vi "AlazarRead.vi"(0 "DeviceIn":i32, 1 "Digitizer Settings":T1={"Digitizer delay (us) "=18.666667, "rf points per line"=4000, "lines per plane"=139, "Samp Rate (Hz)"=100000000.0, "Additional dig delay (us)"=0.0, "Voltage Scale"=0.4, "Pre-Looks"=0, "Offset delay (us)"=2.0, "bits A/D"=0, "Avg Num"=1, "DigTimeOut"=5.0, "Rel Dig Delay"=0.0, "Dig Ch"=0, "LeCroyCluster"={"LeCroy Channels"=[TRUE, FALSE, FALSE, FALSE], "LC read pt offset"=0.0, "Sweep Avg"=FALSE}, "Main Digitizer"=enum."NI Digitizer", "Dig Config"=enum."Single channel", "Digitizer ID Cluster"={"Acqiris/Alazar/SP ID"=[], "NI Instr Handles"=[], "LeCroy VISA"="", "GaGe Handle"={"Handle"=0, "Sample size"=0, "Resolution"=0, "Offset"=0, "Channels"=0, "Boards"=0}, "ATS Ref"="ATS9350", "Acqiris Address"=["PCI::INSTR0"], "ADQRef"=refnum, "adq_cu_ptr"=refnum}, "Trigger Settings"={"Trig Source"=1, "Trig Coupling"=0, "Trig Slope"=0, "Level (mV)"=1500.0}, "Bulk Acq"=FALSE, "Bulk Start Indexes"=[], "Data Ref RF"=refnum, "NI ID/Channel"=[], "Total Dig CH"=1, "Xtra Ann Trig delay (us)"=10.0, "Fix Z Delay?"=FALSE, "One Way Transmission?"=FALSE, "Data Ref Log"=refnum} {"Trigger Settings"."Trig Slope" items=["Positive", "Negative"]; "Trigger Settings"."Level (mV)" format="%.2f"; "Trigger Settings"."Trig Coupling" items=["DC 1 MOhm", "AC 1 MOhm", "DC 50 Ohm", "AC 50 Ohm"]; "Trigger Settings"."Trig Source" items=["Chan 1", "External"]; "Rel Dig Delay" format="%.2f"; "DigTimeOut" format="%.2f"; "Avg Num" min=1; "Offset delay (us)" format="%.2f"; "Additional dig delay (us)" format="%.2f"; "Digitizer delay (us)" format="%.2f"}, 5 "Channel":T5, 9 "RecordIn":u32=1, 11 "ReadSamples":T6) -> (3 "Clock (s)":dbl format="%.2p", 4 "DeviceOut":i32, 6 "TimeStamp (s)":dbl format="%.2p", 8 "Voltage Scaling":dbl, 10 "Presize (s)":dbl format="%.2p", 14 "Binary Data":i16[](array[numeric]), 15 "Return Code":u32)   [LabVIEW 2022 SP3]
doc: "_____AlazarTech, Scope_____\n\nConfigure the capture clock circuitry."
uses:
  C:/AlazarTech/ATS-VI/6.2.0/ATS_ctl/Device_Ctrl.ctl
  ATS_ReadSamples.ctl
  C:/AlazarTech/ATS-VI/6.2.0/ATS_ctl/ATS_Channel.ctl
  -DigitizerRoutines/DigitizerSettings.ctl
  -DigitizerRoutines/DigitizerID.ctl
  -DigitizerRoutines/Digitizer.ctl
  -DigitizerRoutines/DigConfig.ctl
  C:/Windows/System32/ADQAPI_dotNet_helper.dll
panel:
  out "Waveform Graph":i16[](graph)
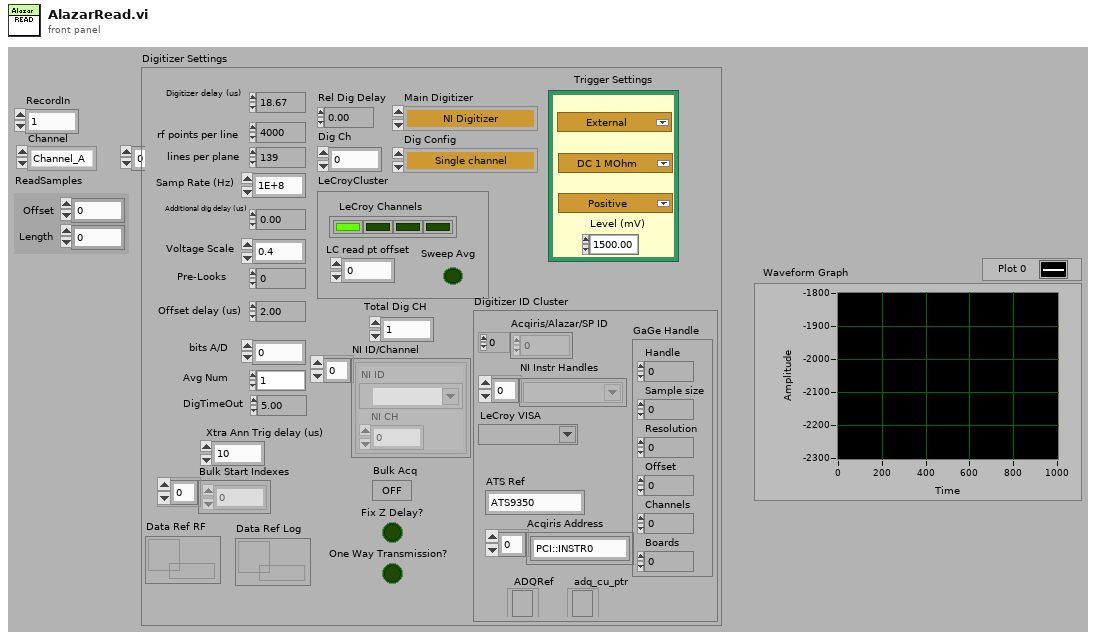
[diagram p1: front panel]
types:
  T1 = typedef "DigitizerSettings.ctl" = cluster{"Digitizer delay (us) ":dbl, "rf points per line":i32, "lines per plane":i32, "Samp Rate (Hz)":dbl, "Additional dig delay (us)":dbl, "Voltage Scale":dbl, "Pre-Looks":i32, "Offset delay (us)":dbl, "bits A/D":i8, "Avg Num":i32, "DigTimeOut":sgl, "Rel Dig Delay":sgl, "Dig Ch":i32, "LeCroyCluster":cluster{"LeCroy Channels":bool[], "LC read pt offset":dbl, "Sweep Avg":bool}, "Main Digitizer":T2, "Dig Config":T3, "Digitizer ID Cluster":T4, "Trigger Settings":cluster{"Trig Source":u16, "Trig Coupling":u16, "Trig Slope":u16, "Level (mV)":dbl}, "Bulk Acq":bool, "Bulk Start Indexes":i32[], "Data Ref RF":refnum<data-value>, "NI ID/Channel":cluster{"NI ID":refnum<k15>, "NI CH":i32}[], "Total Dig CH":i32, "Xtra Ann Trig delay (us)":dbl, "Fix Z Delay?":bool, "One Way Transmission?":bool, "Data Ref Log":refnum<data-value>}
  T2 = typedef "Digitizer.ctl" = enum16{"Acqiris Digitizer", "NI Digitizer", "LeCroy", "GaGe", "AlazarTech", "No Digitizer", "Teledyne"}
  T3 = typedef "DigConfig.ctl" = enum16{"Single channel", "2 Chans w/ 2 Acqiris", "2 Chans w/ 1 Acqiris", "5-CH Pulser New", "5-CH pulser w/ ann array", "5-pass style ann array", "Empty"}
  T4 = typedef "DigitizerID.ctl" = cluster{"Acqiris/Alazar/SP ID":u32[], "NI Instr Handles":refnum<k15>[], "LeCroy VISA":refnum<visa-resource-name>, "GaGe Handle":cluster{"Handle":u32, "Sample size":u32, "Resolution":i32, "Offset":i32, "Channels":u32, "Boards":u32}, "ATS Ref":string, "Acqiris Address":string[], "ADQRef":refnum<k24>, "adq_cu_ptr":refnum<k24>}
  T5 = typedef "ATS_Channel.ctl" = enum16{"Channel_A", "Channel_B", "Channel_C", "Channel_D"}
  T6 = typedef "ATS_ReadSamples.ctl" = cluster{"Offset":i32, "Length":u32}
  T7 = typedef "Device_Ctrl.ctl" = enum16{"Status", "About", "Arm", "ForceTrig", "Abort", "Initialize", "Init (NoPreset)", "Info", "Close", "Calibrate", "SetManually", "LED_ON", "LED_OFF"}
  T8 = typedef "Device_Info.ctl" = cluster{"Handle":u32, "Board":string, "CPLD":string, "MemorySize":u32, "SampleSize":u8, "ID":i32, "High_Memory":bool, "Chan/Board":u8}
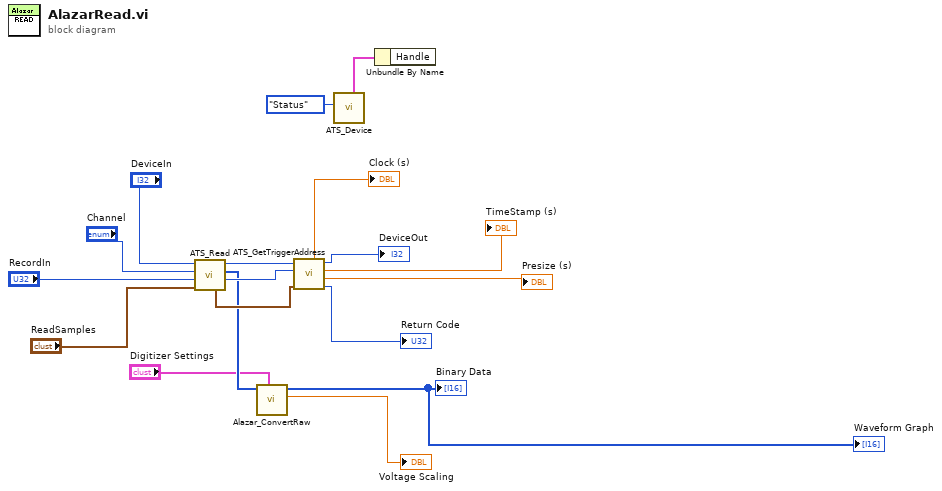
[diagram p0: block diagram]
diagram:
  n1 = call "ATS_Read.vi"("ReadSamples"="ReadSamples", "RecordIn"="RecordIn", "Channel"="Channel", "DeviceIn"="DeviceIn") -> ("RecordOut"=w11:u32, "Buffer"=w4:u16[], "DeviceOut"=w15:i32, "ReadSamples_Out"=w12:T6)  [unwired: 3 in, 1 out]
  n2 = call "Alazar_ConvertRaw.vi"("Digitizer Settings"="Digitizer Settings", "Buffer"=w4) -> ("Voltage multiplier"=→"Voltage Scaling":dbl, "Array"=→"Binary Data" →"Waveform Graph":i16[])  [unwired: 8 in]
  n3 = call "ATS_GetTriggerAddress.vi"("ReadSamples"=w12, "Record"=w11, "DeviceIn"=w15) -> ("Return Code"=→"Return Code":u32, "Presize (s / clk)"=→"Presize (s)":dbl, "TimeStamp (s / clk)"=→"TimeStamp (s)":dbl, "DeviceOut"=→"DeviceOut":i32, "Clock (s / clk)"=→"Clock (s)":dbl)  [unwired: 4 in]
  n4 = call "ATS_Device.vi"("DevCtrl"=Device_Ctrl."Status") -> ("DevInfo"=w17:T8)  [unwired: 4 in, 6 out]
  n5 = Unbundle By Name(w17) -> ()  [unwired: 1 out]
